vi "initialize debug mode.vi"(10 "User Event in":T1, 11 "editor node in":T2) -> (1 "engine":refnum<data-value>, 2 "User Event out":T1, 3 "editor node out":T2)   [LabVIEW 2013, in "user tag bus module editor node.lvclass"]
uses:
  user tag bus module editor node.lvclass
  <vilib>/CEF_TreeControl/Node/NodeRef.ctl
  <vilib>/CEF_TreeControl/Node/NISE_CEF_Node.lvclass
  <vilib>/NI/Tag Bus Data Framework/Configuration Editor/Classes/Engine Parent/Engine Parent Editor Node.lvclass
  <vilib>/CEF_TreeControl/Node/UserEventRef.ctl
  <vilib>/CEF_TreeControl/Controls/EventCluster.ctl
  module/configuration/user tag bus module configuration.lvclass
  <vilib>/NI/Module Execution Interface/Engine Configuration/engine configuration.lvclass
  <vilib>/NI/Tag Bus/tag/Data Type.ctl
  <vilib>/NI/Tag Bus/tag/tag descriptor.lvclass/tag descriptor.ctl
  <vilib>/NI/Tag Bus/tag bus error generator.vi
  <vilib>/NI/Tag Bus/tag/validate default value.vi
  <vilib>/NI/Tag Bus Data Framework/Configuration Editor/Classes/Engine Parent/write engine configuration.vi
  <vilib>/NI/Tag Bus/tag/tag descriptor.lvclass
  <vilib>/CEF_TreeControl/NISE_CEF_TreeControl.lvlib
  <vilib>/NI/Tag Bus Data Framework/Configuration Editor/Classes/Module editor node/module editor node.lvclass
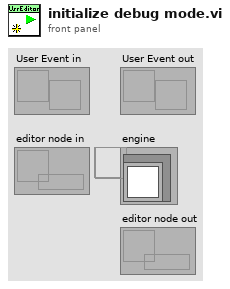
[diagram p1: front panel]
types:
  T1 = typedef "NISE_CEF_Node.lvclass/UserEventRef.ctl" = refnum<user-event>
  T2 = typedef "NISE_CEF_Node.lvclass/NodeRef.ctl" = refnum<data-value>
  T3 = typedef "NISE_CEF_TreeControl.lvlib/EventCluster.ctl" = cluster{"command":string, "data":string}
  T4 = typedef "tag bus.lvlib/tag descriptor.lvclass/Data Type.ctl" = enum16{"Double", "Single", "I64", "I32", "I16", "I8", "U64", "U32", "U16", "U8", "Boolean", "String", "Array of Double", "Array of Single", "Array of I64", "Array of I32", "Array of I16", "Array of I8", "Array of U64", "Array of U32", "Array of U16", "Array of U8", "Array of Boolean", "Array of String"}
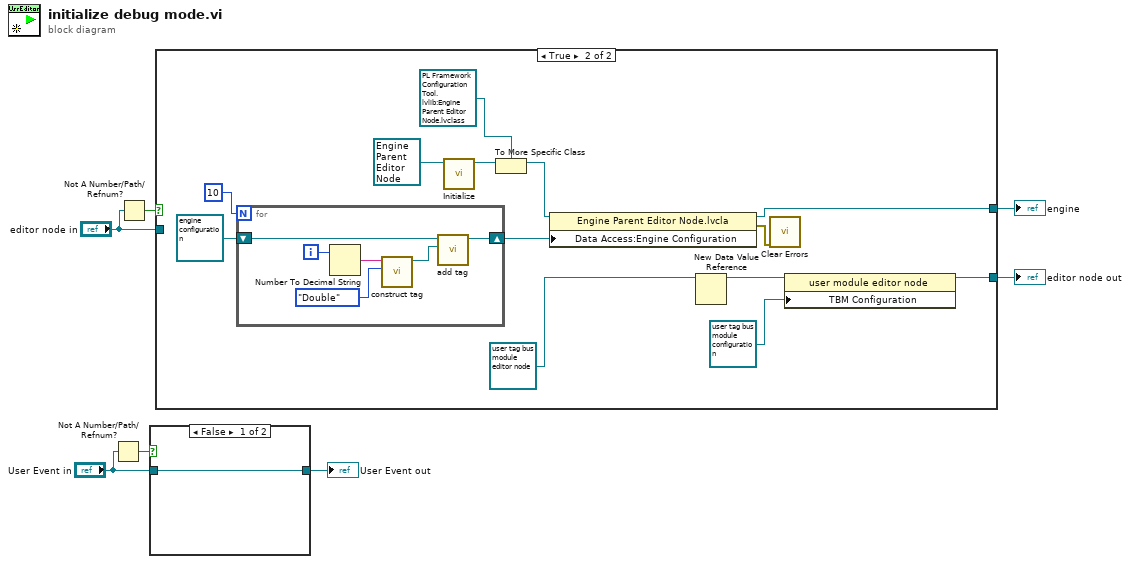
[diagram p0: block diagram]
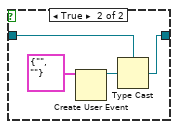
[diagram p2: hidden frame]
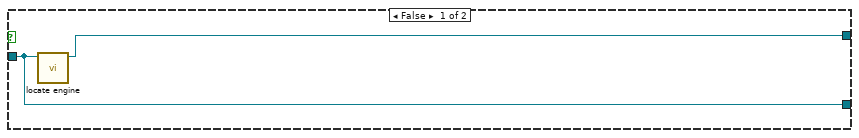
[diagram p3: hidden frame]
diagram:
  n1 = Not A Number/Path/Refnum?(number/path/refnum="User Event in") -> (NaN/Path/Refnum?=w3:bool)
  n2 = Not A Number/Path/Refnum?(number/path/refnum="editor node in") -> (NaN/Path/Refnum?=w4:bool)
  n3 = case shown="False" w3 {
    tunnel: "User Event in" -> [w8 w9]
    tunnel: [w8 w10] -> w1
    frame False {
    }
    frame True {
      n4 = Create User Event(user event datatype=T3 {"command"="", "data"=""} ("event data")) -> (user event=w11:refnum<user-event>)  [unwired: 1 in, 1 out]
      n5 = Type Cast(type=w9, x=w11) -> (*(type *) &x=w10:T1)
    }
  }
  "User Event out" <- w1
  n6 = case shown="True" w4 {
    tunnel: "editor node in" -> [w13 _]
    tunnel: [w13 w27] -> w6
    tunnel: [w14 w19] -> w5
    frame False {
      n7 = call <vilib>:"locate engine.vi"("component"=w13) -> ("engine"=w14:refnum<data-value>)  [unwired: 9 in, 1 out]
    }
    frame True {
      n8 = for {
        N: 10 -> [_]
        shift-right: [w32] -> w17
        shift-left: refnum<class "engine configuration.lvclass"> refnum ("Engine Configuration") -> [w33]
        i -> [w30]
        n9 = Number To Decimal String(number=w30) -> (decimal integer string=w29:string)  [unwired: 1 in]
        n10 = call <vilib>:"construct tag.vi"("data type"=Data_Type."Double", "name"=w29) -> ("system tag out"=w31:refnum<class "tag descriptor.lvclass">)  [unwired: 8 in, 1 out]
        n11 = call <vilib>:"add tag.vi"("tag descriptor"=w31, "engine configuration in"=w33) -> ("engine configuration out"=w32:refnum<class "engine configuration.lvclass">)  [unwired: 8 in, 1 out]
      }
      n12 = call-dynamic "Initialize.vi"("Engine in"=refnum<class "Engine Parent Editor Node.lvclass"> refnum ("PL Framework Configuration Tool.lvlib:Engine Parent Editor Node.lvclass")) -> ("data value reference"=w26:T2)  [unwired: 8 in, 2 out]
      n13 = To More Specific Class(target class=refnum<data-value> refnum ("data value reference"), reference=w26) -> (specific class reference=w25:refnum<data-value>)  [unwired: 1 in, 1 out]
      n14 = property class="Engine Parent Editor Node.lvcla"(reference=w25, "Data Access:Engine Configuration"=w17) -> (reference out=w19:refnum<data-value>, error out=w15:errorcluster)  [unwired: 1 in]
      n15 = New Data Value Reference(data value=refnum<class "user tag bus module editor node.lvclass"> refnum ("tag bus configurable plugin editor node")) -> (data value reference=w23:refnum<data-value>)  [unwired: 1 in, 1 out]
      n16 = call <vilib>:"Clear Errors.vi"("error in (no error)"=w15) -> ()  [unwired: 6 in, 1 out]
      n17 = property class="user module editor node"(reference=w23, "TBM Configuration"=refnum<class "user tag bus module configuration.lvclass"> refnum ("user module configuration")) -> (reference out=w27:refnum<data-value>)  [unwired: 1 in, 1 out]
    }
  }
  "editor node out" <- w6
  "engine" <- w5
